vi "get_unpack_type.vi"(4 "error in":errorcluster, 7 "u":u64) -> (0 "error out":errorcluster, 1 "name":string, 2 "type":u16(ring) items=["Fix"=127, "Null"=192, "False"=194, "True"=195, "Float"=202, "Double"=203, "Uint8"=204, "Uint16"=205, "Uint32"=206, "Uint64"=207, "Int8"=208, "Int16"=209, "Int32"=210, "Int64"=211, "Raw"=218, "Array"=220, "Map"=222, ""=0], 3 "u out":u64)   [LabVIEW 2019, in "msgunpack.lvlib"]
doc: "Returns the type of the next item to be unpacked from the buffer"
uses:
  msgunpack.lvlib
  msgpack.lvlib
  msgpackalt.dll
panel:
  # "msgpack"
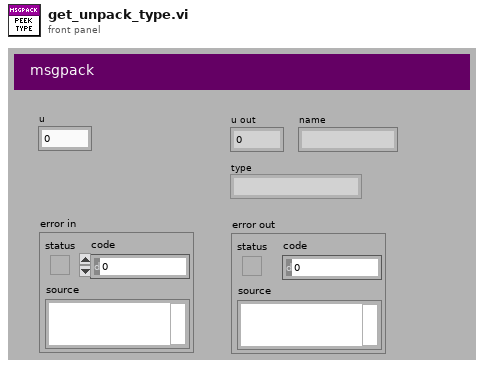
[diagram p1: front panel]
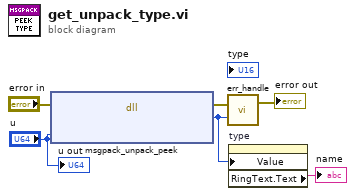
[diagram p0: block diagram]
diagram:
  n1 = dll-call lib="C:/Users/Patrick/Documents/GitHub/Instrument-Framework/lvsrc/SMOs/JSON-RPC-2019/lv-venv/lv.lib/vi.lib/addons/msgpack/msgpackalt.dll" fn="msgpack_unpack_peek"(error in="error in", "p"="u") -> (error out=w5:errorcluster, "return type"=w2:i32)  [unwired: 3 in, 1 out]
  n2 = call "err_handle.vi"("retval"=w2, "error in"=w5) -> ("error out"=→"error out":errorcluster)  [unwired: 1 in]
  n3 = property on="type" class="Ring (strict)"("Value"=w2) -> ("RingText.Text"=→"name":string)  [unwired: 2 in, 2 out]
  "u out" <- "u"
